vi "Regex verify limits.vi"(8 "error in":errorcluster, 11 "input string":string) -> (0 "error out":errorcluster, 2 "Data out":dbl[](array[numeric]), 3 "Valid data":bool)   [LabVIEW 2021]
uses:
  <vilib>/regexp/Match Regular Expression.xnode
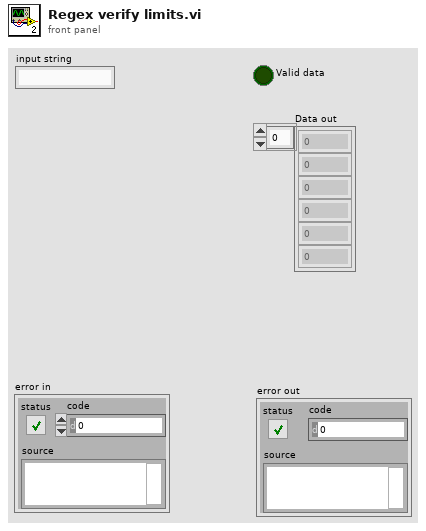
[diagram p1: front panel]
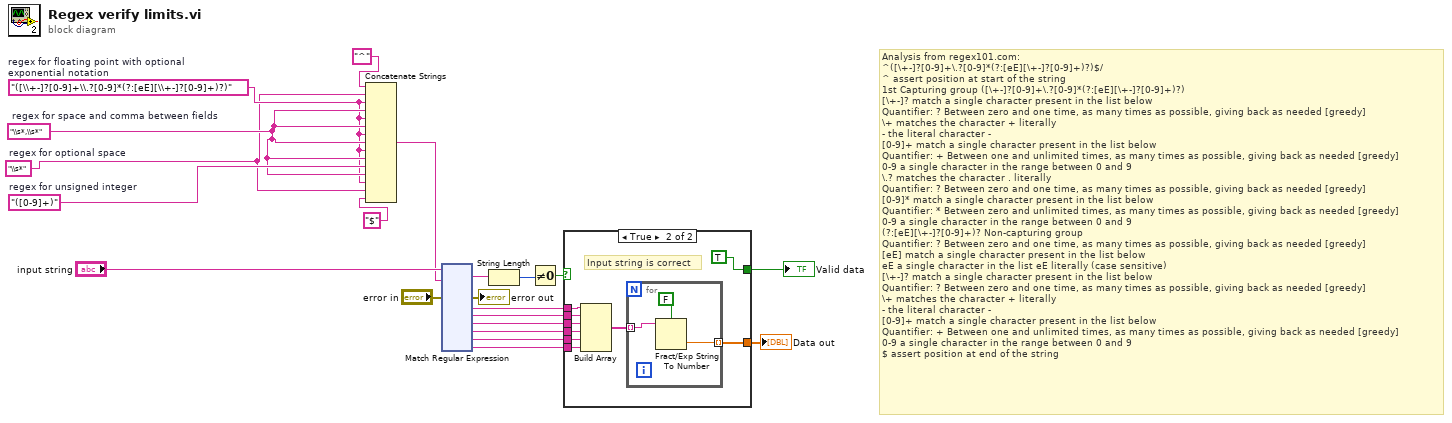
[diagram p0: block diagram]
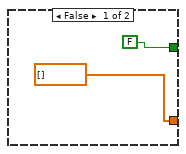
[diagram p2: hidden frame]
diagram:
  w17 = "\\s*"  # regex for optional space
  w20 = "([0-9]+)"  # regex for unsigned integer
  w19 = "\\s*,\\s*"  # regex for space and comma between fields
  w18 = "([\\+-]?[0-9]+\\.?[0-9]*(?:[eE][\\+-]?[0-9]+)?)"  # regex for floating point with optional exponential notation
  # "Analysis from regex101.com:\n^([\\+-]?[0-9]+\\.?[0-9]*(?:[eE][\\+-]?[0-9]+)?)$/\n^ assert position at start of the string\n1st Capturing group ([\\+-]?[0-9]+\\.?[0-9]*(?:[eE][\\+-]?[0-9]+)?)\n[\\+-]? match a single character present in the list below\nQuantifier: ? Between zero and one time, as many times as possible, giving back as needed [greedy]\n\\+ matches the character + literally\n- the literal character -\n[0-9]+ match a single character present in the list below\nQuantifier: + Between one and unlimited times, as many times as possible, giving back as needed [greedy]\n0-9 a single character in the range between 0 and 9\n\\.? matches the character . literally\nQuantifier: ? Between zero and one time, as many times as possible, giving back as needed [greedy]\n[0-9]* match a single character present in the list below\nQuantifier: * Between zero and unlimited times, as many times as possible, giving back as needed [greedy]\n0-9 a single character in the range between 0 and 9\n(?:[eE][\\+-]?[0-9]+)? Non-capturing group\nQuantifier: ? Between zero and one time, as many times as possible, giving back as needed [greedy]\n[eE] match a single character present in the list below\neE a single character in the list eE literally (case sensitive)\n[\\+-]? match a single character present in the list below\nQuantifier: ? Between zero and one time, as many times as possible, giving back as needed [greedy]\n\\+ matches the character + literally\n- the literal character -\n[0-9]+ match a single character present in the list below\nQuantifier: + Between one and unlimited times, as many times as possible, giving back as needed [greedy]\n0-9 a single character in the range between 0 and 9\n$ assert position at end of the string"
  n1 = Concatenate Strings("^", w17, w18, w19, w18, w19, w18, w19, w18, w19, w20, w19, w18, w17, "$") -> (w16:string)
  n2 = xnode "Match Regular Expression"("input string"="input string", "regular expression"=w16, "error in"="error in") -> ("whole match"=w7:string, "error out"=→"error out":errorcluster, "submatch 1"=w13:string, "submatch 2"=w12:string, "submatch 3"=w11:string, "submatch 4"=w10:string, "submatch 5"=w9:string, "submatch 6"=w8:string)  [unwired: 3 in, 3 out]
  n3 = String Length(string=w7) -> (length=w6:i32)
  n4 = Not Equal To 0?(x=w6) -> (x != 0?=w5:bool)
  n5 = case shown="True" w5 {
    tunnel: w13 -> [_ w32]
    tunnel: w12 -> [_ w31]
    tunnel: w11 -> [_ w30]
    tunnel: w10 -> [_ w29]
    tunnel: w9 -> [_ w28]
    tunnel: w8 -> [_ w27]
    tunnel: [dbl[] [] w25] -> w1
    tunnel: [FALSE TRUE] -> w2
    frame False {
    }
    frame True {
      # "Input string is correct"
      n6 = Build Array(w32, w31, w30, w29, w28, w27) -> (w26:string[])
      n7 = for {
        tunnel: w26 -> [w35] mode=indexing
        tunnel: [w33] -> w25 mode=indexing
        n8 = Fract/Exp String To Number(use system decimal point (T)=FALSE, string=w35) -> (number=w33:dbl)  [unwired: 2 in, 1 out]
      }
    }
  }
  "Valid data" <- w2
  "Data out" <- w1
